vi "Enumerate VISA.vi"(8 "error in (no error)":errorcluster) -> (0 "error out":errorcluster, 3 "Ports":T1(array[cluster]))   [LabVIEW 2022 SP3]
uses:
  <vilib>/Utility/config.llb/Read Key (I32).vi
  <vilib>/Utility/config.llb/Read Key (String).vi
  <vilib>/Utility/config.llb/NI_LVConfig.lvlib
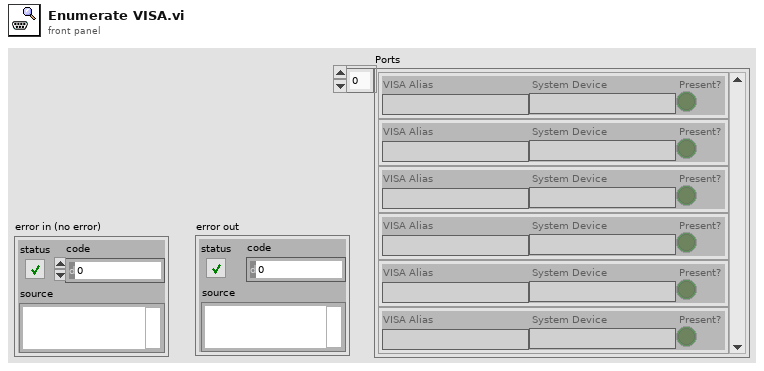
[diagram p1: front panel]
types:
  T1 = cluster{"VISA Alias":string, "System Device":string, "Present?":bool}[]
  T2 = typedef "NI_LVConfig.lvlib/Config Data RefNum.ctl" = refnum<k1>
  T3 = cluster{"value":string, "value":string, "file or folder exists?":bool}
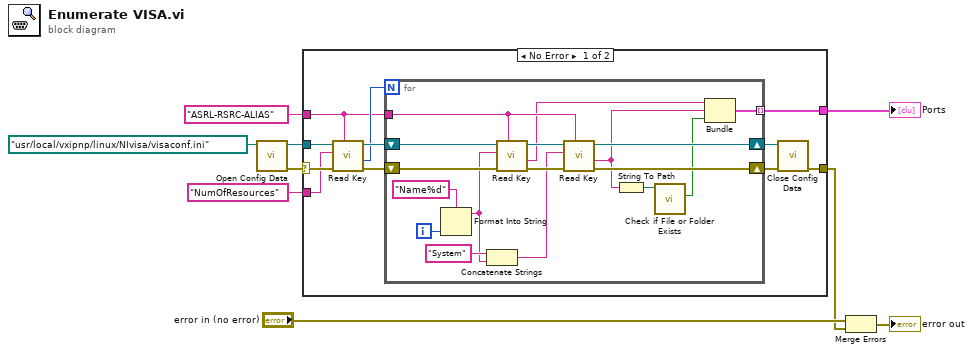
[diagram p0: block diagram]
diagram:
  n1 = call <vilib>:"Open Config Data.vi"("configuration file path"=path "/usr/local/vxipnp/linux/NIvisa/visaconf.ini") -> ("error out"=w7:errorcluster, "refnum"=w8:T2)  [unwired: 8 in, 1 out]
  n2 = case shown="No Error" w7 {
    selector: w7 -> [w20 w38]
    tunnel: w8 -> [w19 _]
    tunnel: "ASRL-RSRC-ALIAS" ("section") -> [w14 _]
    tunnel: "NumOfResources" ("section") -> [w18 _]
    tunnel: [w13 _] -> w4
    tunnel: [w10 w38] -> w2
    frame No Error {
      n3 = call-poly <vilib>:"Read Key.vi"("section"=w14, "error in (no error)"=w20, "key"=w18, "refnum"=w19) -> ("error out"=w16:errorcluster, "value"=w15:i32, "refnum out"=w17:T2)  [unwired: 4 in, 1 out]
      n4 = for {
        N: w15 -> [_]
        shift-right: [w27] -> w12
        shift-left: w17 -> [w37]
        shift-right: [w28] -> w11
        shift-left: w16 -> [w36]
        tunnel: w14 -> [w26]
        tunnel: [w21] -> w13 mode=indexing
        i -> [w34]
        n5 = Format Into String(format string="Name%d", w34) -> (resulting string=w32:string)  [unwired: 2 in, 1 out]
        n6 = Concatenate Strings("System" ("string"), w32) -> (w29:string)
        n7 = call-poly <vilib>:"Read Key.vi"("section"=w26, "error in (no error)"=w36, "key"=w32, "refnum"=w37) -> ("error out"=w31:errorcluster, "value"=w24:string, "refnum out"=w30:T2)  [unwired: 4 in, 1 out]
        n8 = call-poly <vilib>:"Read Key.vi"("section"=w26, "error in (no error)"=w31, "key"=w29, "refnum"=w30) -> ("error out"=w28:errorcluster, "value"=w23:string, "refnum out"=w27:T2)  [unwired: 4 in, 1 out]
        n9 = String To Path(string=w23) -> (path=w25:path)
        n10 = call <vilib>:"Check if File or Folder Exists.vi"("path"=w25) -> ("file or folder exists?"=w22:bool)  [unwired: 8 in, 2 out]
        n11 = Bundle("value"=w24, "value"=w23, "file or folder exists?"=w22) -> (w21:T3)  [unwired: 1 in]
      }
      n12 = call <vilib>:"Close Config Data.vi"("error in (no error)"=w11, "refnum"=w12) -> ("error out"=w10:errorcluster)  [unwired: 8 in, 1 out]
    }
    frame Error {
    }
  }
  "Ports" <- w4
  n13 = Merge Errors("error in (no error)", w2) -> (→"error out":errorcluster)
